vi "Read NI 9422 - Counter Driven Output.vi"(8 "error in":errorcluster, 11 "NI 9422 in":refnum<class "NI 9422.lvclass">) -> (0 "error out":errorcluster, 1 "channel settings":T2[](array[typedef]), 2 "drive from slot":T1, 3 "NI 9422 out":refnum<class "NI 9422.lvclass">)   [LabVIEW 2017, in "NI 9422.lvclass"]
uses:
  NI 9422.lvclass
  Channel Classes/Counter Driven Output Channel/Counter Driven State.ctl
  Channel Classes/Counter Driven Output Channel/Counter Driven Output Channel.lvclass
  Mode Classes/Controls/counter driven output channel settings.ctl
  Scan Engine Scripting.lvlib
  Mode Classes/Counter Driven Output Mode/Drive from Slot.ctl
  Mode Classes/Counter Driven Output Mode/Counter Driven Output Mode.lvclass
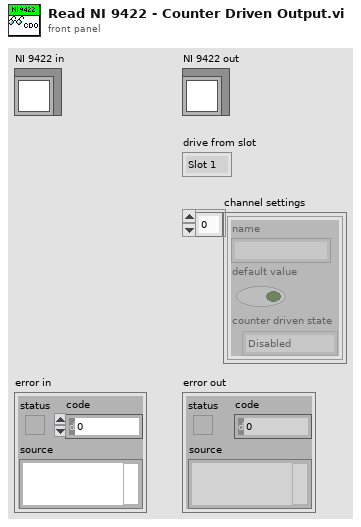
[diagram p1: front panel]
types:
  T1 = typedef "Scan Engine Scripting.lvlib/Counter Driven Output Mode.lvclass/Drive from Slot.ctl" = enum16{"Slot 1", "Slot 2", "Slot 3", "Slot 4", "Slot 5", "Slot 6", "Slot 7", "Slot 8"}
  T2 = typedef "Scan Engine Scripting.lvlib/counter driven output channel settings.ctl" = cluster{"name":string, "default value":bool, "counter driven state":T3}
  T3 = typedef "Scan Engine Scripting.lvlib/Counter Driven Output Channel.lvclass/Counter Driven State.ctl" = enum16{"Disabled", "Enabled"}
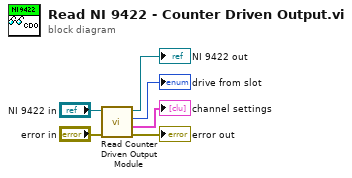
[diagram p0: block diagram]
diagram:
  n1 = call-dynamic "Read Counter Driven Output Module.vi"("error in"="error in", "module in"="NI 9422 in") -> ("error out"=→"error out":errorcluster, "channel settings"=→"channel settings":T2[], "drive from slot"=→"drive from slot":T1, "module out"=→"NI 9422 out":refnum<class "NI 9422.lvclass">)  [unwired: 6 in]
